vi "Process Messages.vi"(8 "error in (no error)":errorcluster, 11 "Mixer in":refnum<class "Transport.lvclass">) -> (0 "error out":errorcluster, 3 "Mixer out":refnum<class "Transport.lvclass">)   [LabVIEW 2020, in "Transport.lvclass"]
uses:
  Transport.lvclass
  Transport.lvclass/Transport.ctl
  Packed Libraries/Messaging.lvlibp
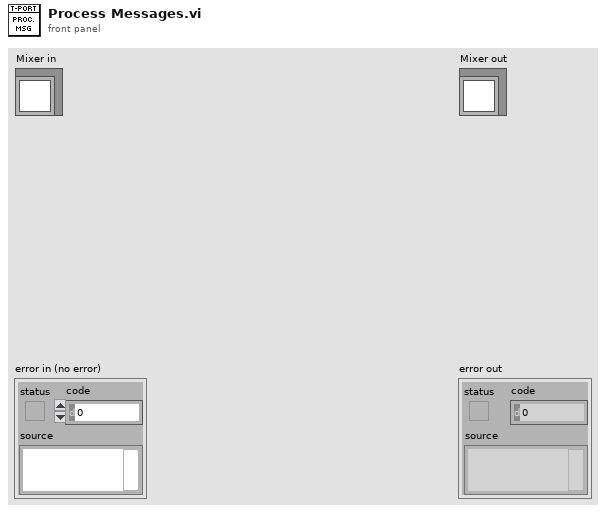
[diagram p1: front panel]
types:
  T1 = typedef "Messaging.lvlibp/Message Cluster.ctl" = cluster{"Event":string, "Source":string, "Target":string, "Data":variant}
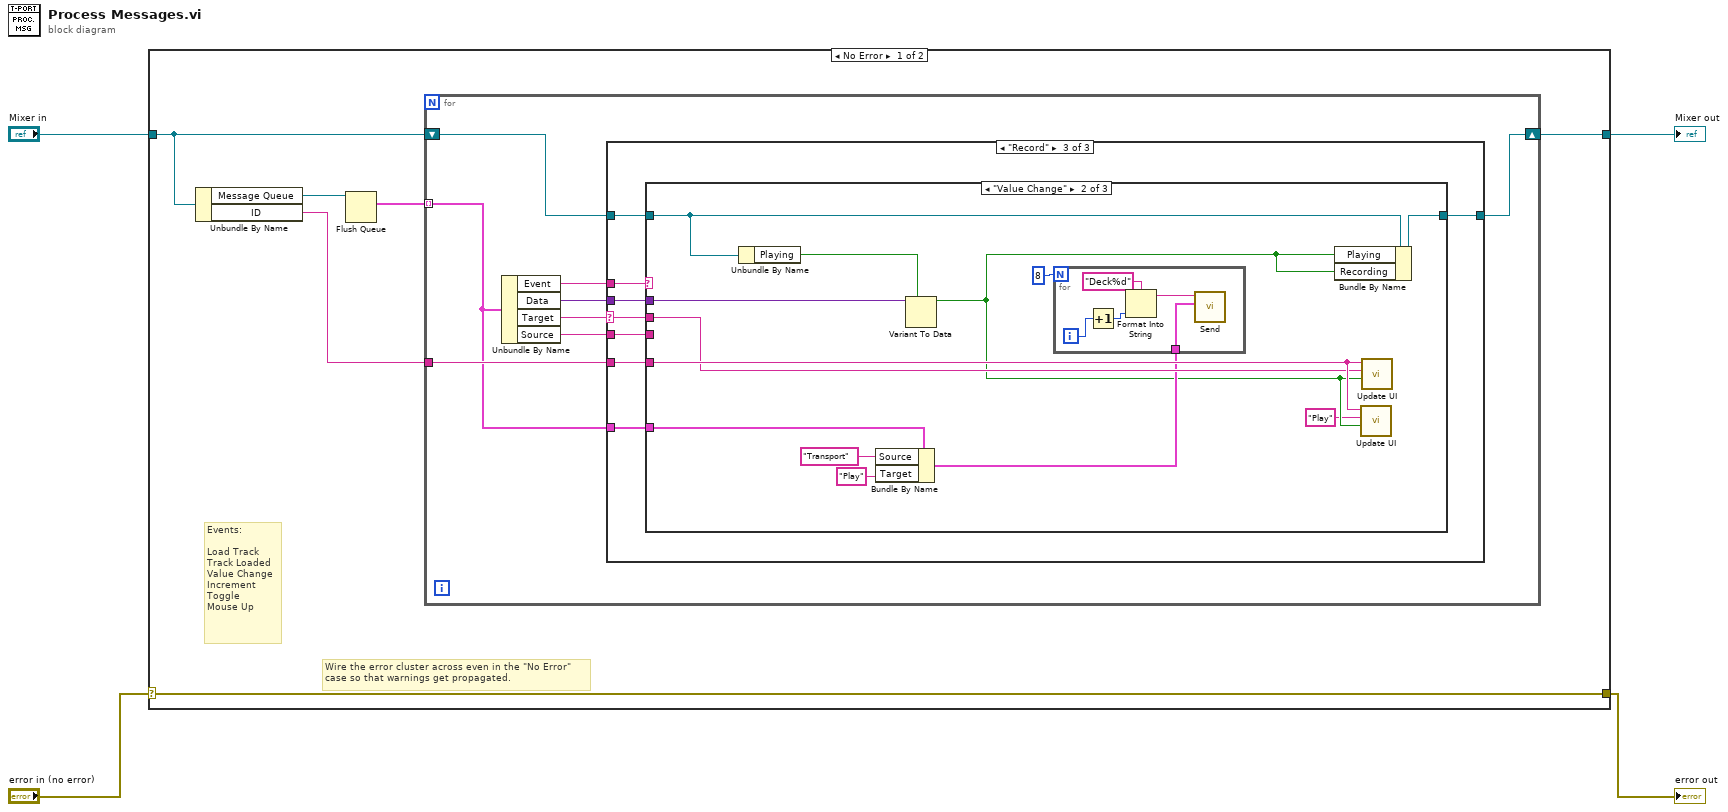
[diagram p0: block diagram]
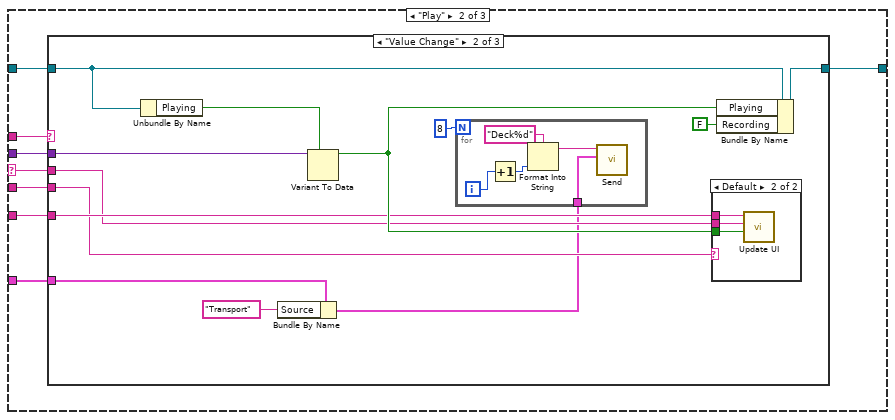
[diagram p3: hidden frame]
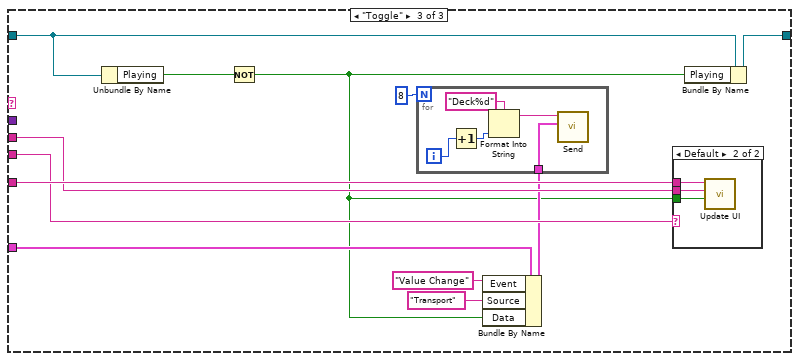
[diagram p6: hidden frame]
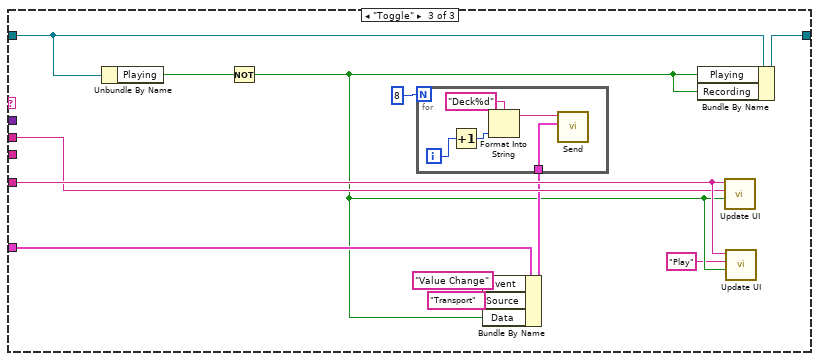
[diagram p9: hidden frame]
diagram:
  n1 = case shown="No Error" "error in (no error)" {
    selector: "error in (no error)" -> [w10 w115]
    tunnel: [w10 w115] -> w2
    tunnel: [w5 w114] -> w1
    tunnel: "Mixer in" -> [w9 w114]
    frame No Error {
      # "Events:\n\nLoad Track\nTrack Loaded\nValue Change\nIncrement\nToggle\nMouse Up"
      # "Wire the error cluster across even in the \"No Error\"\ncase so that warnings get propagated."
      n2 = Unbundle By Name(w9) -> ("Message Queue"=w8:refnum<queue>, "ID"=w6:string)
      n3 = Flush Queue(queue=w8) -> (remaining elements=w7:T1[])  [unwired: 1 in, 2 out]
      n4 = for {
        shift-right: [w17] -> w5
        shift-left: w9 -> [w18]
        tunnel: w7 -> [w11] mode=indexing
        tunnel: w6 -> [w12]
        n5 = Unbundle By Name(w11) -> ("Event"=w14:string, "Data"=w15:variant, "Target"=w16:string, "Source"=w13:string)
        n6 = case shown="\"Record\"" w16 {
          selector: w16 -> [_ w22 w72]
          tunnel: w18 -> [w19 w25 w75]
          tunnel: [w19 w26 w76] -> w17
          tunnel: w15 -> [_ w24 w74]
          tunnel: w14 -> [_ w27 w77]
          tunnel: w13 -> [_ w23 w73]
          tunnel: w12 -> [_ w21 w71]
          tunnel: w11 -> [_ w20 w70]
          frame Default {
          }
          frame "Play" {
            n7 = case shown="\"Value Change\"" w27 {
              tunnel: [w28 w38 w60] -> w26
              tunnel: w25 -> [w28 w39 w61]
              tunnel: w24 -> [_ w40 _]
              tunnel: w23 -> [_ w34 w57]
              tunnel: w22 -> [_ w35 w58]
              tunnel: w21 -> [_ w36 w59]
              tunnel: w20 -> [_ w32 w55]
              frame Default {
              }
              frame "Value Change" {
                n8 = Unbundle By Name(w39) -> ("Playing"=w41:bool)
                n9 = Bundle By Name(cluster=w32, "Source"="Transport") -> (w30:T1)
                n10 = Variant To Data(type=w41, Variant=w40) -> (data=w37:bool)  [unwired: 1 in, 1 out]
                n11 = for {
                  N: 8 -> [_]
                  tunnel: w30 -> [w46]
                  i -> [w45]
                  n12 = Increment(x=w45) -> (x+1=w44:i32)
                  n13 = Format Into String(format string="Deck%d", w44) -> (resulting string=w42:string)  [unwired: 2 in, 1 out]
                  n14 = call "Send.vi"("Message"=w46, "Queue Name"=w42) -> ()  [unwired: 9 in, 1 out]
                }
                n15 = case shown="Default" w34 {
                  tunnel: w36 -> [_ w49]
                  tunnel: w35 -> [_ w48]
                  tunnel: w37 -> [_ w47]
                  frame "UI" {
                  }
                  frame Default {
                    n16 = call "Update UI.vi"("Data"=w47, "Target"=w48, "ID"=w49) -> ()  [unwired: 8 in, 1 out]
                  }
                }
                n17 = Bundle By Name(cluster=w39, "Playing"=w37, "Recording"=FALSE) -> (w38:refnum<class "Transport.lvclass">)
              }
              frame "Toggle" {
                n18 = Unbundle By Name(w61) -> ("Playing"=w52:bool)
                n19 = Not(x=w52) -> (.not. x?=w50:bool)
                n20 = Bundle By Name(cluster=w55, "Event"="Value Change", "Source"="Transport", "Data"=w50) -> (w53:T1)
                n21 = for {
                  N: 8 -> [_]
                  tunnel: w53 -> [w66]
                  i -> [w65]
                  n22 = Increment(x=w65) -> (x+1=w64:i32)
                  n23 = Format Into String(format string="Deck%d", w64) -> (resulting string=w62:string)  [unwired: 2 in, 1 out]
                  n24 = call "Send.vi"("Message"=w66, "Queue Name"=w62) -> ()  [unwired: 9 in, 1 out]
                }
                n25 = case shown="Default" w57 {
                  tunnel: w59 -> [_ w69]
                  tunnel: w58 -> [_ w68]
                  tunnel: w50 -> [_ w67]
                  frame "UI" {
                  }
                  frame Default {
                    n26 = call "Update UI.vi"("Data"=w67, "Target"=w68, "ID"=w69) -> ()  [unwired: 8 in, 1 out]
                  }
                }
                n27 = Bundle By Name(cluster=w61, "Playing"=w50) -> (w60:refnum<class "Transport.lvclass">)
              }
            }
          }
          frame "Record" {
            n28 = case shown="\"Value Change\"" w77 {
              tunnel: [w78 w88 w107] -> w76
              tunnel: w75 -> [w78 w89 w108]
              tunnel: w74 -> [_ w90 _]
              tunnel: w73 -> [_ _ _]
              tunnel: w72 -> [_ w86 w105]
              tunnel: w71 -> [_ w87 w106]
              tunnel: w70 -> [_ w84 w103]
              frame Default {
              }
              frame "Value Change" {
                n29 = Unbundle By Name(w89) -> ("Playing"=w91:bool)
                n30 = Bundle By Name(cluster=w84, "Source"="Transport", "Target"="Play" ("Event")) -> (w82:T1)
                n31 = Variant To Data(type=w91, Variant=w90) -> (data=w81:bool)  [unwired: 1 in, 1 out]
                n32 = for {
                  N: 8 -> [_]
                  tunnel: w82 -> [w96]
                  i -> [w95]
                  n33 = Increment(x=w95) -> (x+1=w94:i32)
                  n34 = Format Into String(format string="Deck%d", w94) -> (resulting string=w92:string)  [unwired: 2 in, 1 out]
                  n35 = call "Send.vi"("Message"=w96, "Queue Name"=w92) -> ()  [unwired: 9 in, 1 out]
                }
                n36 = Bundle By Name(cluster=w89, "Playing"=w81, "Recording"=w81) -> (w88:refnum<class "Transport.lvclass">)
                n37 = call "Update UI.vi"("Data"=w81, "Target"="Play", "ID"=w87) -> ()  [unwired: 8 in, 1 out]
                n38 = call "Update UI.vi"("Data"=w81, "Target"=w86, "ID"=w87) -> ()  [unwired: 8 in, 1 out]
              }
              frame "Toggle" {
                n39 = Unbundle By Name(w108) -> ("Playing"=w100:bool)
                n40 = Not(x=w100) -> (.not. x?=w98:bool)
                n41 = Bundle By Name(cluster=w103, "Event"="Value Change", "Source"="Transport", "Data"=w98) -> (w101:T1)
                n42 = for {
                  N: 8 -> [_]
                  tunnel: w101 -> [w113]
                  i -> [w112]
                  n43 = Increment(x=w112) -> (x+1=w111:i32)
                  n44 = Format Into String(format string="Deck%d", w111) -> (resulting string=w109:string)  [unwired: 2 in, 1 out]
                  n45 = call "Send.vi"("Message"=w113, "Queue Name"=w109) -> ()  [unwired: 9 in, 1 out]
                }
                n46 = Bundle By Name(cluster=w108, "Playing"=w98, "Recording"=w98) -> (w107:refnum<class "Transport.lvclass">)
                n47 = call "Update UI.vi"("Data"=w98, "Target"=w105, "ID"=w106) -> ()  [unwired: 8 in, 1 out]
                n48 = call "Update UI.vi"("Data"=w98, "Target"="Play", "ID"=w106) -> ()  [unwired: 8 in, 1 out]
              }
            }
          }
        }
      }
    }
    frame Error {
    }
  }
  "error out" <- w2
  "Mixer out" <- w1
